vi "SyncLoopHandler.vi"(8 "error in (no error)":errorcluster, 10 "LoopProperties":refnum<class "SyncPluginBase.lvclass">, 11 "PXI_MultiTrig in":refnum<class "PXI_MultiTrig.lvclass">) -> (0 "error out":errorcluster, 3 "PXI_MultiTrig out":refnum<class "PXI_MultiTrig.lvclass">)   [LabVIEW 2018, in "SyncPlugins.lvlib" / "PXI_MultiTrig.lvclass"]
uses:
  PXI_MultiTrig.lvclass
  X:/Projects/PMUCal/Modules/Sync/SyncPlugins/SyncPluginBase/SyncPluginBase.lvclass
  SyncPluginBase/SyncPluginBase.lvclass
  SyncPluginBase/SyncPluginBase.lvclass/SyncPluginBase.ctl
  SyncPluginBase/Accessors/Write Run.vi
  SyncPluginBase/Accessors/Write Monitor Loop.vi
  SyncPluginBase/Accessors/Write Locked.vi
  SyncPluginBase/Accessors/Read Locked.vi
  SyncPluginBase/Accessors/Read Run.vi
  SyncPluginBase/Accessors/Read LostLock.vi
  Typedefs/clClocks.ctl
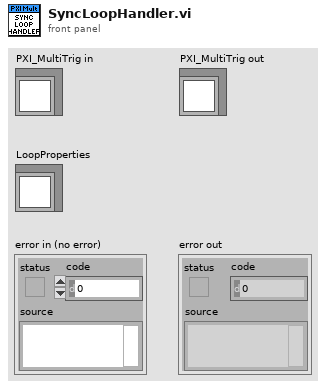
[diagram p1: front panel]
types:
  T1 = typedef "SyncPlugins.lvlib/PXI_MultiTrig.lvclass/clClocks.ctl" = cluster{"Name":string, "RefClk":string, "ClkTerminal":string, "Frequency":dbl, "DutyCycle":dbl, "ClkType":string, "Initiated":bool, "TrigTime":bool, "Delay":dbl}
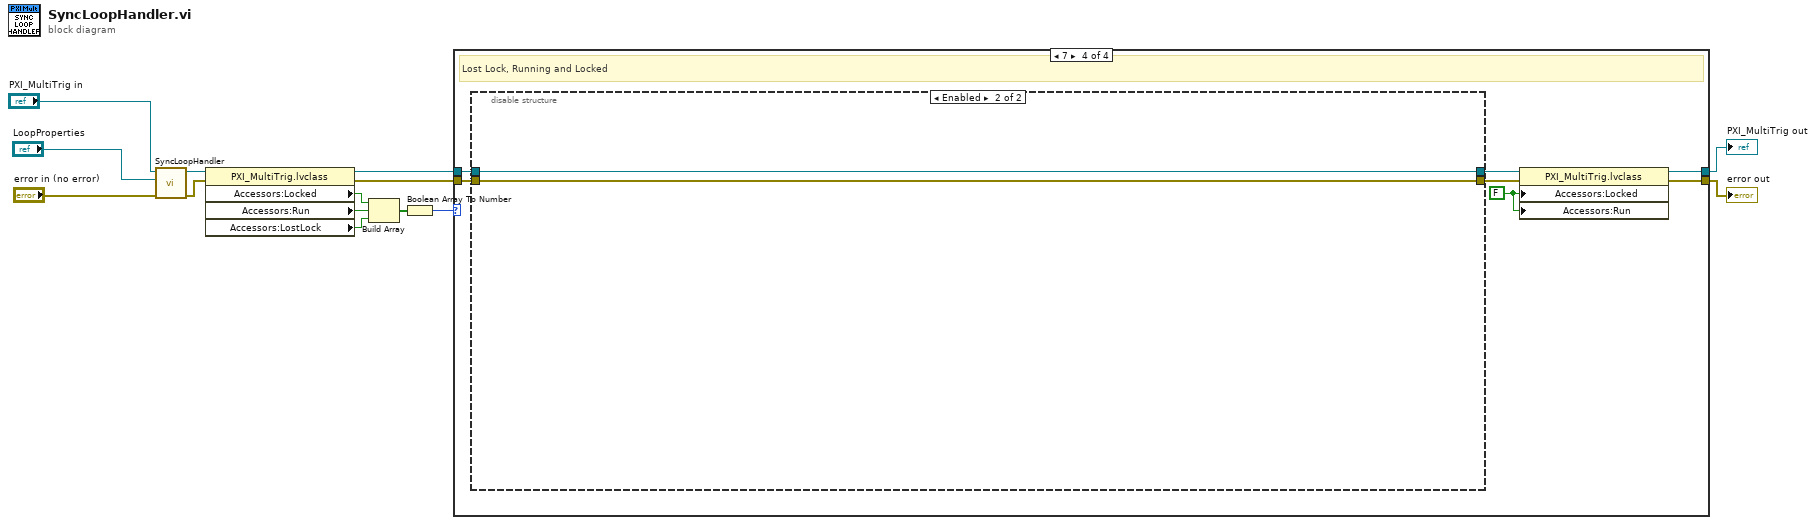
[diagram p0: block diagram]
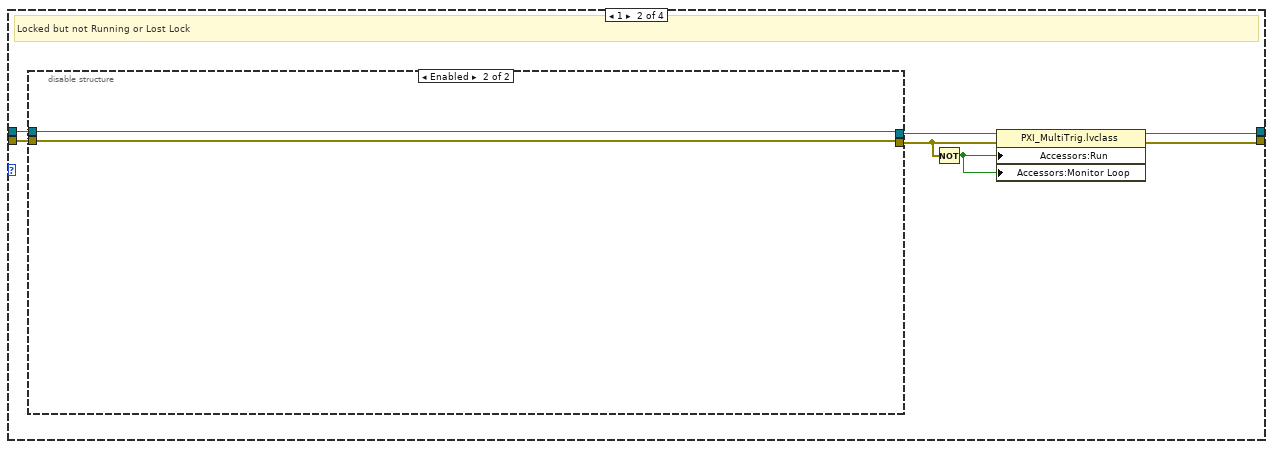
[diagram p3: hidden frame]
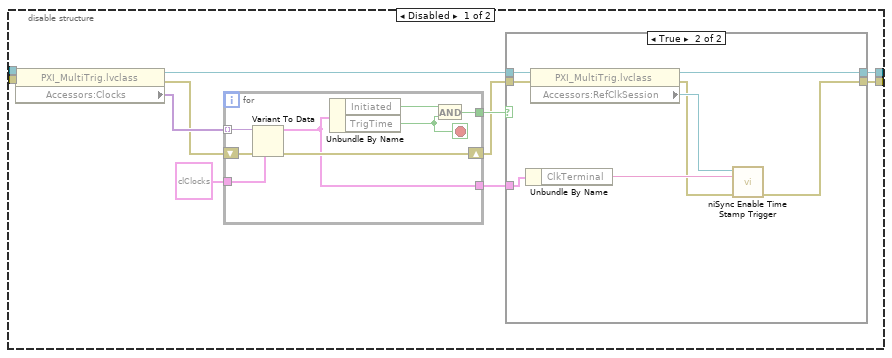
[diagram p4: hidden frame]
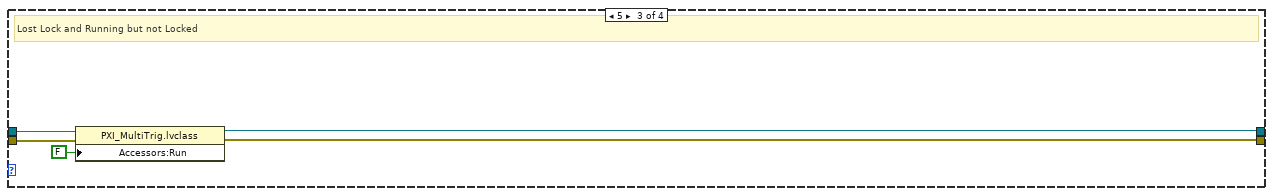
[diagram p6: hidden frame]
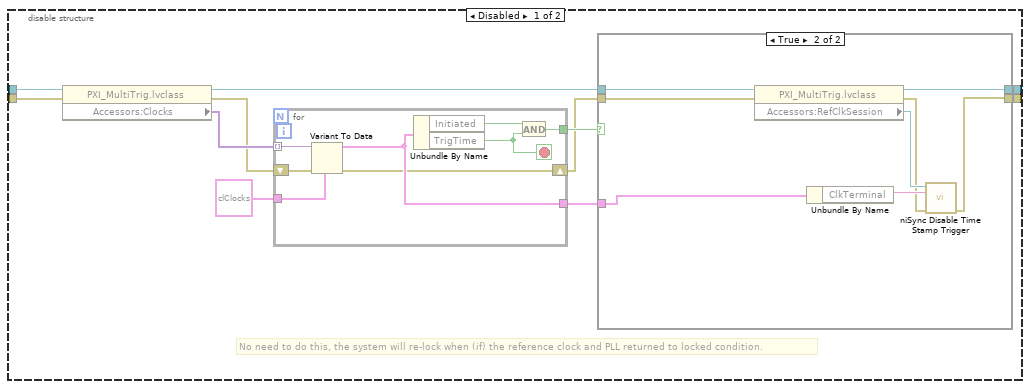
[diagram p7: hidden frame]
diagram:
  n1 = call-parent "SyncLoopHandler.vi"("error in (no error)"="error in (no error)", "LoopProperties"="LoopProperties", "SyncPluginBase in"="PXI_MultiTrig in") -> ("error out"=w11:errorcluster, "SyncPluginBase out"=w14:refnum<class "PXI_MultiTrig.lvclass">)  [unwired: 7 in]
  n2 = property class="PXI_MultiTrig.lvclass"(reference=w14, error in=w11) -> (reference out=w5:refnum<class "PXI_MultiTrig.lvclass">, error out=w4:errorcluster, "Accessors:Locked"=w10:bool, "Accessors:Run"=w8:bool, "Accessors:LostLock"=w9:bool)
  n3 = Build Array(w10, w8, w9) -> (w7:bool[])
  n4 = Boolean Array To Number(Boolean array=w7) -> (number=w6:u32)
  n5 = case shown="7" w6 {
    tunnel: w5 -> [w16 w23 w59 w65]
    tunnel: w4 -> [w15 w22 w58 w66]
    tunnel: [w16 w20 w56 w61] -> w3
    tunnel: [w15 w19 w55 w60] -> w2
    frame 0, Default {
      # "Default, do nothing"
    }
    frame 1 {
      # "Locked but not Running or Lost Lock"
      n6 = disable-structure shown="Enabled" {
        disable-tunnel: w23 -> [w34 w54]
        disable-tunnel: w22 -> [w29 w53]
        disable-tunnel: [w28 w54] -> w21
        disable-tunnel: [w27 w53] -> w18
        frame Disabled {
          n7 = property class="PXI_MultiTrig.lvclass"(reference=w34, error in=w29) -> (reference out=w32:refnum<class "PXI_MultiTrig.lvclass">, error out=w26:errorcluster, "Accessors:Clocks"=w31:variant[])
          n8 = for {
            tunnel: w31 -> [w49] mode=indexing
            tunnel: [w45] -> w30
            tunnel: [w51] -> w33
            shift-right: [w47] -> w25
            shift-left: w26 -> [w48]
            tunnel: T1 {"Name"="", "RefClk"="/PXI1Slot7/PFI1", "ClkTerminal"="PXI_Star4", "Frequency"=0.0, "DutyCycle"=0.0, "ClkType"="", "Initiated"=FALSE, "TrigTime"=FALSE, "Delay"=0.0} ("clClocks") -> [w46]
            stop <- w50 stop-if-true
            n9 = Variant To Data(error in=w48, type=w46, Variant=w49) -> (data=w45:T1, error out=w47:errorcluster)
            n10 = Unbundle By Name(w45) -> ("Initiated"=w52:bool, "TrigTime"=w50:bool)
            n11 = And(x=w52, y=w50) -> (x .and. y?=w51:bool)
          }
          n12 = case shown="True" w33 {
            tunnel: w30 -> [_ w41]
            tunnel: w32 -> [w36 w44]
            tunnel: w25 -> [w35 w42]
            tunnel: [w35 w37] -> w27
            tunnel: [w36 w38] -> w28
            frame False {
            }
            frame True {
              n13 = Unbundle By Name(w41) -> ("ClkTerminal"=w43:string)
              n14 = property class="PXI_MultiTrig.lvclass"(reference=w44, error in=w42) -> (reference out=w38:refnum<class "PXI_MultiTrig.lvclass">, error out=w39:errorcluster, "Accessors:RefClkSession"=w40:refnum<k15>)
              n15 = call <instrlib>:"niSync Enable Time Stamp Trigger.vi"("error in (no error)"=w39, "terminal"=w43, "instrument handle"=w40) -> ("error out"=w37:errorcluster)  [unwired: 6 in, 1 out]
            }
          }
        }
        frame Enabled {
        }
      }
      n16 = Not(x=w18) -> (.not. x?=w17:bool)
      n17 = property class="PXI_MultiTrig.lvclass"(reference=w21, error in=w18, "Accessors:Run"=w17, "Accessors:Monitor Loop"=w17) -> (reference out=w20:refnum<class "PXI_MultiTrig.lvclass">, error out=w19:errorcluster)
    }
    frame 5 {
      # "Lost Lock and Running but not Locked"
      n18 = property class="PXI_MultiTrig.lvclass"(reference=w59, error in=w58, "Accessors:Run"=FALSE ("Run")) -> (reference out=w56:refnum<class "PXI_MultiTrig.lvclass">, error out=w55:errorcluster)
    }
    frame 7 {
      w62 = FALSE
      # "Lost Lock, Running and Locked"
      n19 = disable-structure shown="Enabled" {
        disable-tunnel: w66 -> [w77 w96]
        disable-tunnel: w65 -> [w76 w97]
        disable-tunnel: [w71 w97] -> w64
        disable-tunnel: [w70 w96] -> w63
        frame Disabled {
          # "No need to do this, the system will re-lock when (if) the reference clock and PLL returned to locked condition."
          n20 = property class="PXI_MultiTrig.lvclass"(reference=w76, error in=w77) -> (reference out=w75:refnum<class "PXI_MultiTrig.lvclass">, error out=w68:errorcluster, "Accessors:Clocks"=w72:variant[])
          n21 = for {
            tunnel: w72 -> [w95] mode=indexing
            tunnel: [w90] -> w73
            tunnel: [w93] -> w74
            tunnel: T1 {"Name"="", "RefClk"="/PXI1Slot7/PFI1", "ClkTerminal"="PXI_Star4", "Frequency"=0.0, "DutyCycle"=0.0, "ClkType"="", "Initiated"=FALSE, "TrigTime"=FALSE, "Delay"=0.0} ("clClocks") -> [w91]
            shift-right: [w88] -> w67
            shift-left: w68 -> [w89]
            stop <- w92 stop-if-true
            n22 = Variant To Data(error in=w89, type=w91, Variant=w95) -> (data=w90:T1, error out=w88:errorcluster)
            n23 = Unbundle By Name(w90) -> ("Initiated"=w94:bool, "TrigTime"=w92:bool)
            n24 = And(x=w94, y=w92) -> (x .and. y?=w93:bool)
          }
          n25 = case shown="True" w74 {
            tunnel: w73 -> [_ w84]
            tunnel: w75 -> [w79 w87]
            tunnel: w67 -> [w78 w85]
            tunnel: [w78 w80] -> w70
            tunnel: [w79 w81] -> w71
            frame False {
            }
            frame True {
              n26 = property class="PXI_MultiTrig.lvclass"(reference=w87, error in=w85) -> (reference out=w81:refnum<class "PXI_MultiTrig.lvclass">, error out=w82:errorcluster, "Accessors:RefClkSession"=w83:refnum<k15>)
              n27 = Unbundle By Name(w84) -> ("ClkTerminal"=w86:string)
              n28 = call <instrlib>:"niSync Disable Time Stamp Trigger.vi"("error in (no error)"=w82, "terminal"=w86, "instrument handle"=w83) -> ("error out"=w80:errorcluster)  [unwired: 6 in, 1 out]
            }
          }
        }
        frame Enabled {
        }
      }
      n29 = property class="PXI_MultiTrig.lvclass"(reference=w64, error in=w63, "Accessors:Locked"=w62, "Accessors:Run"=w62) -> (reference out=w61:refnum<class "PXI_MultiTrig.lvclass">, error out=w60:errorcluster)
    }
  }
  "error out" <- w2
  "PXI_MultiTrig out" <- w3
